vi "Controller - FGV - Root Actor Enqueuer.vi"(7 "Action":T1=enum."Get", 8 "error in":errorcluster, 10 "Actor's Enqueuer":refnum<class "Message Enqueuer.lvclass">) -> (0 "error out":errorcluster, 2 "Root Enqueuer":refnum<class "Message Enqueuer.lvclass">)   [LabVIEW 2023, in "Controller.lvlib" / "Controller.lvclass"]
uses:
  Controller.lvclass
  Controller - Ctrl - FGV - Action.ctl
  <vilib>/ActorFramework/Message Enqueuer/Message Enqueuer.lvclass
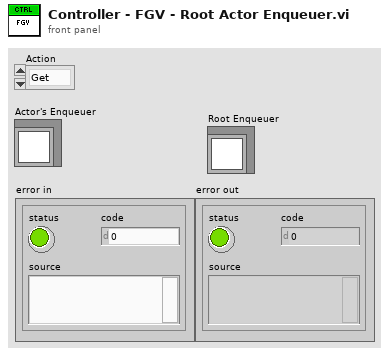
[diagram p1: front panel]
types:
  T1 = typedef "Controller.lvlib/Controller.lvclass/Controller - Ctrl - FGV - Action.ctl" = enum16{"Int", "Get"}
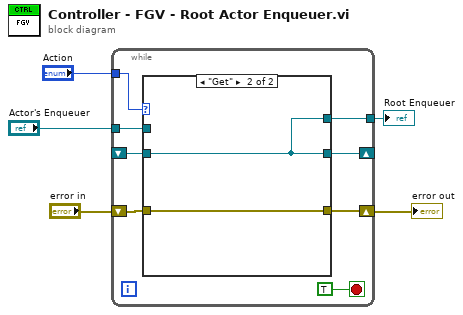
[diagram p0: block diagram]
diagram:
  n1 = while {
    tunnel: "Action" -> [w13]
    shift-right: [w11] -> w3
    shift-left: "error in" -> [w12]
    shift-right: [w9] -> _
    shift-left: _ -> [w7]
    tunnel: "Actor's Enqueuer" -> [w8]
    tunnel: [w6] -> w1
    stop <- TRUE stop-if-true
    n2 = case shown="\"Get\"" w13 {
      tunnel: w12 -> [w15 w17]
      tunnel: [w15 w17] -> w11
      tunnel: [w14 w16] -> w9
      tunnel: w8 -> [w14 _]
      tunnel: w7 -> [_ w16]
      tunnel: [_ w16] -> w6
      frame "Int", Default {
      }
      frame "Get" {
      }
    }
  }
  "error out" <- w3
  "Root Enqueuer" <- w1
